vi "tsa_AR Predictor (F).vi"(0 "Response signal":dbl[](array[numeric]) format="%.2f", 1 "not R matrix":bool, 3 "order":i32=4, 4 "block size":i32=1000) -> (5 "R Matrix":dbl[][](array[numeric]) format="%.2f", 7 "F Vector":dbl[](array[numeric]) format="%.2f")   [LabVIEW 2017, in "NI_AALPro.lvlib"]
uses:
  <vilib>/Analysis/NI_AALPro.lvlib
  <vilib>/Analysis/baseanly.llb/A x Vector.vi
  <vilib>/Analysis/baseanly.llb/Real A x B.vi
  <vilib>/Analysis/7linalg.llb/Create Special Real Matrix.vi
  <vilib>/Analysis/NI_AALBase.lvlib
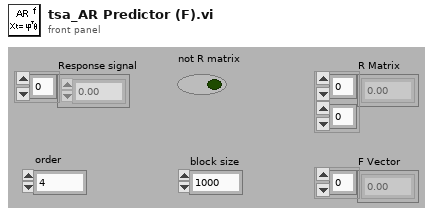
[diagram p1: front panel]
types:
  T1 = enum32{"Identity", "Diagonal", "Toepliz", "Vandermonde", "Companion"}
  T2 = typedef "NI_Matrix.lvlib/RealMatrix.ctl" = dbl[][]
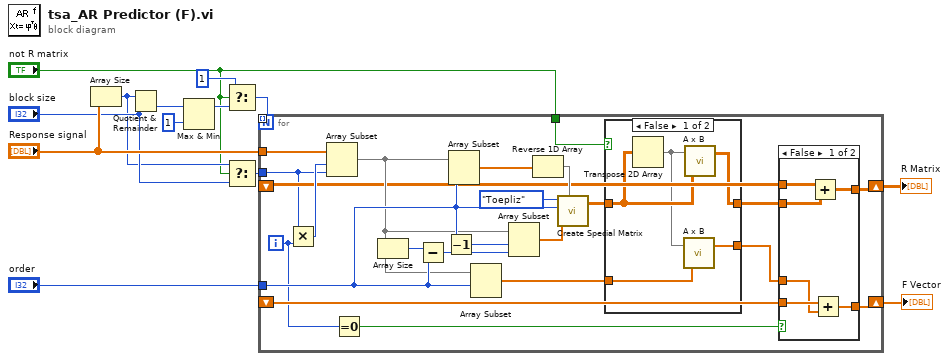
[diagram p0: block diagram]
diagram:
  n1 = Array Size(array="Response signal") -> (size(s)=w3:i32)
  n2 = Quotient & Remainder(x=w3, y="block size") -> (floor(x/y)=w11:i32)  [unwired: 1 out]
  n3 = Max & Min(x=w11, y=1) -> (max(x,y)=w6:i32)  [unwired: 1 out]
  n4 = Select(t=1, s="not R matrix", f=w6) -> (s? t:f=w7:i32)
  n5 = Select(t=w3, s="not R matrix", f="block size") -> (s? t:f=w5:i32)
  n6 = for {
    N: w7 -> [w15]
    tunnel: "Response signal" -> [w31]
    tunnel: "order" -> [w29]
    tunnel: w5 -> [w14]
    shift-right: [w26] -> w9
    shift-left: _ -> [w21]
    shift-right: [w24] -> w8
    shift-left: _ -> [w25]
    tunnel: "not R matrix" -> [w16]
    tunnel: [w15] -> _ mode=indexing
    i -> [w23]
    n7 = Multiply(x=w14, y=w23) -> (x*y=w27:i32)
    n8 = Array Subset(array=w31, index=w27, length=w14) -> (w28:dbl[])
    n9 = Equal To 0?(x=w23) -> (x = 0?=w22:bool)
    n10 = Array Size(array=w28) -> (size(s)=w37:i32)
    n11 = Subtract(x=w37, y=w29) -> (x-y=w32:i32)
    n12 = Decrement(x=w29) -> (x-1=w30:i32)
    n13 = Array Subset(array=w28, length=w29) -> (w35:dbl[])  [unwired: 1 in]
    n14 = Array Subset(array=w28, index=w29) -> (w19:dbl[])  [unwired: 1 in]
    n15 = Array Subset(array=w28, index=w30, length=w32) -> (w33:dbl[])
    n16 = Reverse 1D Array(array=w35) -> (reversed array=w34:dbl[])
    n17 = call-poly <vilib>:"Create Special Matrix.vi"("matrix type"=T1."Toepliz", "matrix size"=w29, "Input Vector1"=w33, "Input Vector2"=w34) -> ("Special Matrix"=w20:T2)  [unwired: 1 in, 1 out]
    n18 = case shown="False" w16 {
      tunnel: w20 -> [w42 w44]
      tunnel: w19 -> [w40 w43]
      tunnel: [w39 w43] -> w18
      tunnel: [w38 w44] -> w17
      frame False {
        n19 = Transpose 2D Array(2D array=w42) -> (transposed array=w41:T2)
        n20 = call-poly <vilib>:"A x B.vi"("Vector"=w40, "A"=w41) -> ("A x Vector"=w39:dbl[])  [unwired: 1 out]
        n21 = call-poly <vilib>:"A x B.vi"("B"=w42, "A"=w41) -> ("A x B"=w38:T2)  [unwired: 1 out]
      }
      frame True {
      }
    }
    n22 = case shown="False" w22 {
      tunnel: w21 -> [w50 _]
      tunnel: [w49 w52] -> w26
      tunnel: w17 -> [w48 w52]
      tunnel: w25 -> [w47 _]
      tunnel: [w46 w51] -> w24
      tunnel: w18 -> [w45 w51]
      frame False {
        n23 = Add(x=w50, y=w48) -> (x+y=w49:T2)
        n24 = Add(x=w47, y=w45) -> (x+y=w46:dbl[])
      }
      frame True {
      }
    }
  }
  "R Matrix" <- w9
  "F Vector" <- w8
